vi "Stop All Manger SubPanels.vi"(8 "error in (no error)":errorcluster, 11 "CIF_UI in":refnum<class "CIF_Manager_UI.lvclass">) -> (0 "error out":errorcluster)   [LabVIEW 2021, in "CIF_Manager_UI.lvclass"]
uses:
  CIF_Manager_UI.lvclass
  CIF_Manager_UI.lvclass/CIF_Manager_UI.ctl
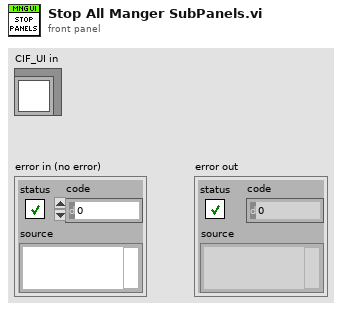
[diagram p1: front panel]
types:
  T1 = typedef "CIF_Manager_UI.lvclass/Manager Subpanel Map.ctl" = map{T2, T3}
  T2 = typedef "CIF_Manager_UI.lvclass/Manager Subpanel Type.ctl" = enum16{"System", "Errors", "Channel", "Plugin"}
  T3 = typedef "CIF_UI.lvclass/Subpanel Data.ctl" = cluster{"VI Reference":refnum<vi>, "Plugin Subpanel Events":T4}
  T4 = typedef "CIF_UI.lvclass/Plugin Subpanel Events.ctl" = cluster{"Plugin Shutdown":refnum<user-event>}
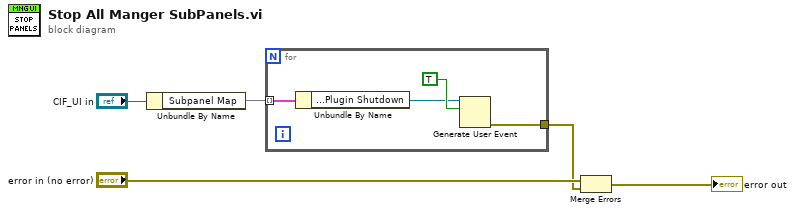
[diagram p0: block diagram]
diagram:
  n1 = Unbundle By Name("CIF_UI in") -> ("Subpanel Map"=w3:T1)
  n2 = for {
    tunnel: w3 -> [w7] mode=indexing
    tunnel: [w8] -> w1
    n3 = Unbundle By Name(w7) -> ("SubPanel Data.Plugin Subpanel Events.Plugin Shutdown"=w6:refnum<user-event>)
    n4 = Generate User Event(user event=w6, event data cluster=TRUE ("event data")) -> (error out=w8:errorcluster)  [unwired: 2 in, 1 out]
  }
  n5 = Merge Errors("error in (no error)", w1) -> (→"error out":errorcluster)
